vi "Send.vi"(9 "Priority?":bool, 10 "Msg Strategy":refnum<class "Msg Strategy.lvclass">, 11 "Queue Msg Type Strategy in":refnum<class "Queue Msg Type Strategy.lvclass">) -> (0 "error out":errorcluster)   [LabVIEW 2021, in "jettl.lvlib" / "Msg Type Strategy.lvlib" / "Queue Msg Type Strategy.lvclass"]
uses:
  Queue Msg Type Strategy.lvclass
  Msg Strategy/Msg Strategy.lvclass
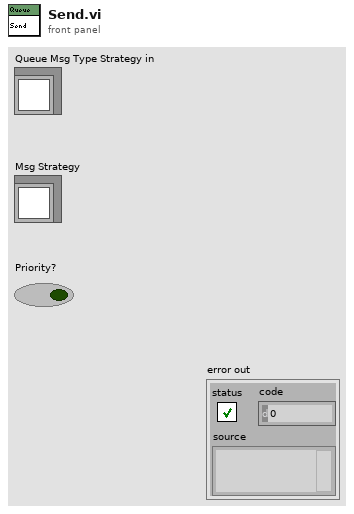
[diagram p1: front panel]
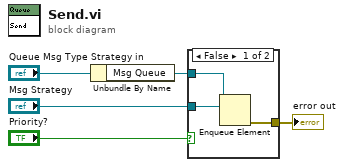
[diagram p0: block diagram]
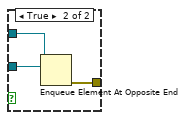
[diagram p2: hidden frame]
diagram:
  n1 = Unbundle By Name("Queue Msg Type Strategy in") -> ("Msg Queue"=w1:refnum<queue>)
  n2 = case shown="False" "Priority?" {
    tunnel: [w8 w10] -> w4
    tunnel: w1 -> [w7 w9]
    tunnel: "Msg Strategy" -> [w6 w11]
    frame False {
      n3 = Enqueue Element(queue=w7, element=w6) -> (error out=w8:errorcluster)  [unwired: 2 in, 2 out]
    }
    frame True {
      n4 = Enqueue Element At Opposite End(queue=w9, element=w11) -> (error out=w10:errorcluster)  [unwired: 2 in, 2 out]
    }
  }
  "error out" <- w4
